vi "sub_resample_and_demodulate.vi"(4 "packet_arr":cdb[][](array[numeric]), 5 "Rx IQ Sampling\nRate [s/sec]":dbl, 6 "error in (no error)":errorcluster, 9 "PSK Init Parameters":T2) -> (0 "error out":errorcluster, 1 "recovered complex waveform":T1[](array[typedef]) {"Y" format="%.3f"; "dt" format="%^.2e"; "t0" format="%.4f"}, 2 "output bit stream":i8[][](array[numeric]), 3 "Sync Found":bool)   [LabVIEW 2011]
uses:
  <vilib>/addons/Modulation/Analog/controls/Complex Data Waveform.ctl
  <vilib>/addons/Modulation/niAMT.lvlib
  <vilib>/addons/Modulation/niDMT.lvlib
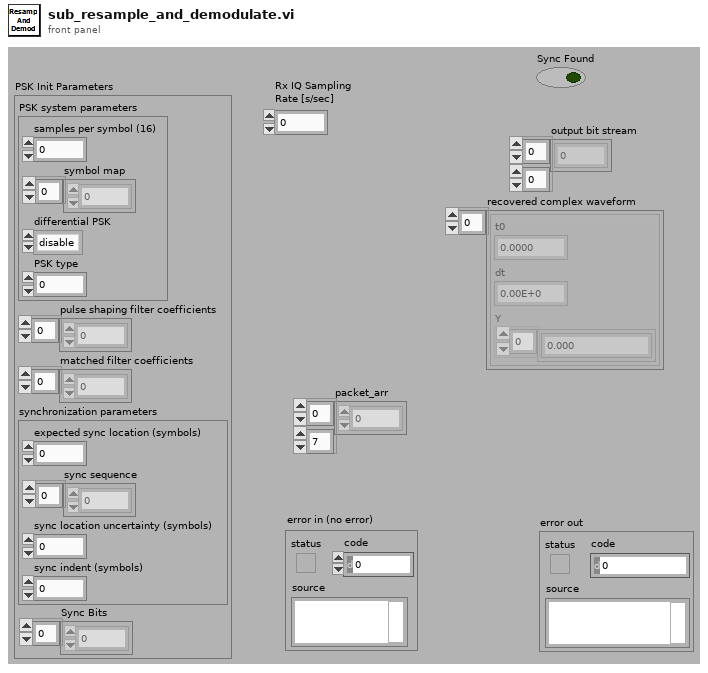
[diagram p1: front panel]
types:
  T1 = typedef "niAMT.lvlib/Complex Data Waveform.ctl" = cluster{"t0":dbl, "dt":dbl, "Y":cdb[]}
  T2 = cluster{"PSK system parameters":cluster{"samples per symbol (16)":i32, "symbol map":cdb[], "differential PSK":enum16{"disable", "enable"}, "PSK type":u16}, "pulse shaping filter coefficients":dbl[], "matched filter coefficients":dbl[], "synchronization parameters":cluster{"expected sync location (symbols)":i32, "sync sequence":cdb[], "sync location uncertainty (symbols)":i32, "sync indent (symbols)":i32}, "Sync Bits":i8[]}
  T3 = cluster{"samples per symbol (16)":i32, "symbol map":cdb[], "differential PSK":enum16{"disable", "enable"}, "PSK type":u16}
  T4 = cluster{"expected sync location (symbols)":i32, "sync sequence":cdb[], "sync location uncertainty (symbols)":i32, "sync indent (symbols)":i32}
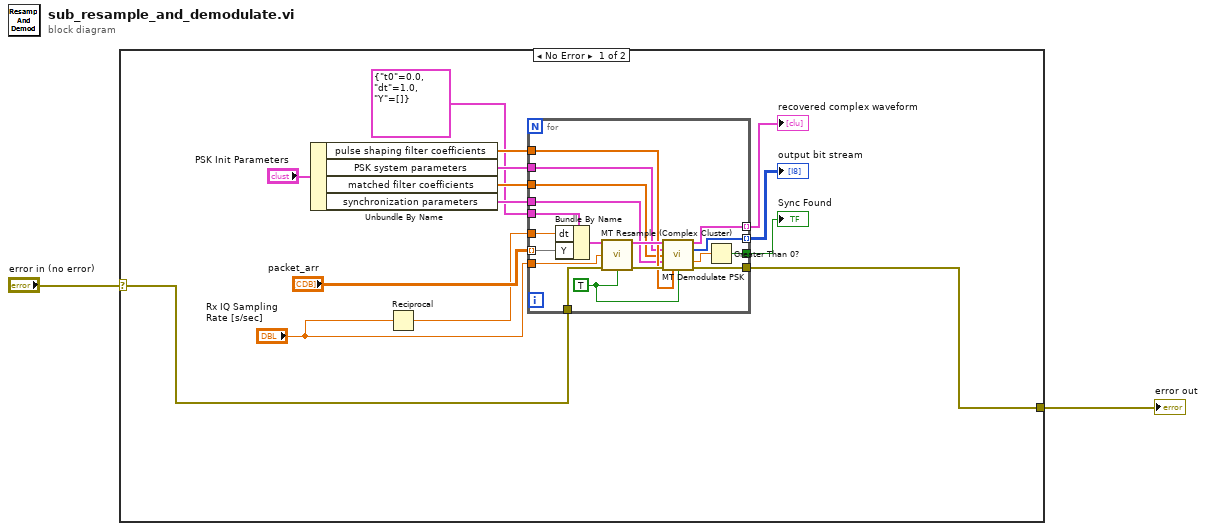
[diagram p0: block diagram]
diagram:
  n1 = case shown="No Error" "error in (no error)" {
    selector: "error in (no error)" -> [w3 w35]
    tunnel: [w13 w35] -> w2
    frame No Error {
      n2 = Unbundle By Name("PSK Init Parameters") -> ("pulse shaping filter coefficients"=w8:dbl[], "PSK system parameters"=w11:T3, "matched filter coefficients"=w10:dbl[], "synchronization parameters"=w9:T4)
      n3 = Reciprocal(x="Rx IQ Sampling\nRate [s/sec]") -> (1/x=w5:dbl)
      n4 = for {
        tunnel: "packet_arr" -> [w17] mode=indexing
        tunnel: "Rx IQ Sampling\nRate [s/sec]" -> [w32]
        tunnel: w8 -> [w31]
        tunnel: w10 -> [w30]
        tunnel: w11 -> [w29]
        tunnel: [w28] -> w15 mode=indexing
        tunnel: w9 -> [w27]
        tunnel: [w25] -> w16
        tunnel: [w24] -> w13
        tunnel: [w22] -> w7 mode=indexing
        tunnel: w5 -> [w21]
        tunnel: T1 {"t0"=0.0, "dt"=1.0, "Y"=[]} ("input complex waveform") -> [w20]
        tunnel: w3 -> [w18]
        w23 = TRUE ("reset? (T)")
        n5 = Bundle By Name(cluster=w20, "dt"=w21, "Y"=w17) -> (w19:T1)
        n6 = call <vilib>:"MT Resample (Complex Cluster).vi"("input complex waveform"=w19, "desired sample rate (Hz)"=w32, "error in (no error)"=w18, "reset? (T)"=w23) -> ("output complex waveform"=w34:T1, "error out"=w33:errorcluster)  [unwired: 10 in]
        n7 = call <vilib>:"MT Demodulate PSK.vi"("input complex waveform"=w34, "PSK system parameters"=w29, "matched filter coefficients"=w30, "synchronization parameters"=w27, "error in (no error)"=w33, "pulse shaping filter coefficients"=w31, "reset? (T)"=w23) -> ("recovered complex waveform"=w22:T1, "output bit stream"=w28:i8[], "sync found index (symbols)"=w26:dbl, "error out"=w24:errorcluster)  [unwired: 4 in, 1 out]
        n8 = Greater Than 0?(x=w26) -> (x > 0?=w25:bool)
      }
      "Sync Found" <- w16
      "output bit stream" <- w15
      "recovered complex waveform" <- w7
    }
    frame Error {
    }
  }
  "error out" <- w2
